vi "ActionVIOnCompile.vi"(8 "error in":errorcluster, 11 "Device Item Ref in":T1 format="%.0x") -> (0 "error out":errorcluster)   [LabVIEW 2024, in "AIM ARINC 429 System Explorer.lvlib"]
uses:
  AIM ARINC 429 System Explorer.lvlib
  <vilib>/NI VeriStand/Custom Device API/Custom Device API.lvlib
  Includes/AIM ARINC 429 Engine.lvlibp/Engine/Custom Device/Inline Execution Unit Compiled Information.ctl
  Includes/AIM ARINC 429 Engine.lvlibp/Engine/Custom Device/Asynchronous Execution Unit Compiled Information.ctl
  Includes/AIM ARINC 429 Engine.lvlibp/Engine/Custom Device/Compiled.Settings.ctl
  Shared/Constants.vi
  Shared/AIM ARINC 429 Shared.lvlib
  Includes/AIM ARINC 429 Engine.lvlibp/Engine/Implementation/Execution Unit Factory/Execution Unit Factory.lvclass
  Includes/AIM ARINC 429 Engine.lvlibp/Engine/Implementation/Shared Resources Factory/Shared Resources Factory.lvclass
  Includes/AIM ARINC 429 Engine.lvlibp/Engine/Interfaces/Execution Unit Factory/Execution Unit Factory.lvclass
  Includes/AIM ARINC 429 Engine.lvlibp/Engine/Interfaces/Shared Resources Factory/Shared Resources Factory.lvclass
  Includes/AIM ARINC 429 Engine.lvlibp/1abvi3w/vi.lib/NI VeriStand/Custom Device API/Data Reference.ctl
  Includes/AIM ARINC 429 Engine.lvlibp/1abvi3w/vi.lib/NI VeriStand/Custom Device API/Block Data Reference.ctl
  <vilib>/NI VeriStand/Custom Device API/Set Item Property (Variant).vi
  <vilib>/NI VeriStand/Custom Device API/Custom Device Item Ref.ctl
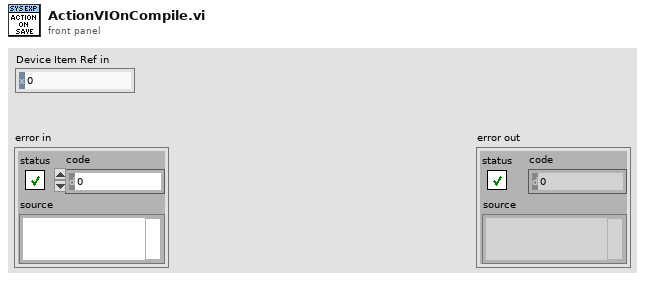
[diagram p1: front panel]
types:
  T1 = typedef "Custom Device API.lvlib/Custom Device Item Ref.ctl" = u64
  T2 = typedef "AIM ARINC 429 System Explorer.lvlibp/Custom Device API.lvlib/Custom Device Item Ref.ctl" = u64
  T3 = typedef "AIM ARINC 429 Engine.lvlibp/Custom Device.lvlib/Compiled.Settings.ctl" = cluster{"Name":string, "Inline Execution Unit Compiled Information":T4[], "Asynchronous Execution Unit Compiled Information":T7[], "Flattened Shared Resources":string}
  T4 = typedef "AIM ARINC 429 Engine.lvlibp/Custom Device.lvlib/Inline Execution Unit Compiled Information.ctl" = cluster{"Flattened Execution Unit":string, "Incoming Buffer":dbl[], "Outgoing Buffer":dbl[], "Incoming Data References":T5[], "Outgoing Data References":T6[]}
  T5 = typedef "AIM ARINC 429 Engine.lvlibp/Custom Device API.lvlib/Data Reference.ctl" = i32
  T6 = typedef "AIM ARINC 429 Engine.lvlibp/Custom Device API.lvlib/Block Data Reference.ctl" = cluster{"Data Reference":T5, "Offset":u64, "Length":u64}
  T7 = typedef "AIM ARINC 429 Engine.lvlibp/Custom Device.lvlib/Asynchronous Execution Unit Compiled Information.ctl" = cluster{"Flattened Execution Unit":string, "Incoming Channel Group Name":string, "Outgoing Channel Group Name":string, "ReadWrite Channel Group Name":string}
  T8 = typedef "Custom Device API.lvlib/Custom Device Item Info.ctl" = cluster{"Name":string, "Is Channel":bool, "GUID":string, "Is Waveform":bool}
  T9 = typedef "AIM ARINC 429 Engine.lvlibp/Interfaces.lvlib/Execution Unit Information.ctl" = cluster{"Execution Unit":refnum<class "Execution Unit.lvclass">, "Incoming Channels":T10[], "Outgoing Channels":T10[], "ReadWrite Channels":T10[]}
  T10 = typedef "AIM ARINC 429 Engine.lvlibp/Custom Device API.lvlib/Custom Device Item Ref.ctl" = u64
  T11 = typedef "AIM ARINC 429 Shared.lvlib/Inline Execution Unit Compiled Information.ctl" = cluster{"Flattened Execution Unit":string, "Incoming Buffer":dbl[], "Outgoing Buffer":dbl[], "Incoming Data References":T12[], "Outgoing Data References":T13[]}
  T12 = typedef "Custom Device API.lvlib/Data Reference.ctl" = i32
  T13 = typedef "Custom Device API.lvlib/Block Data Reference.ctl" = cluster{"Data Reference":T12, "Offset":u64, "Length":u64}
  T14 = typedef "AIM ARINC 429 Shared.lvlib/Asynchronous Execution Unit Compiled Information.ctl" = cluster{"Flattened Execution Unit":string, "Incoming Channel Group Name":string, "Outgoing Channel Group Name":string, "ReadWrite Channel Group Name":string}
  T15 = cluster{"Compiled Grouped Asynchronous Execution Units":T14[]}[]
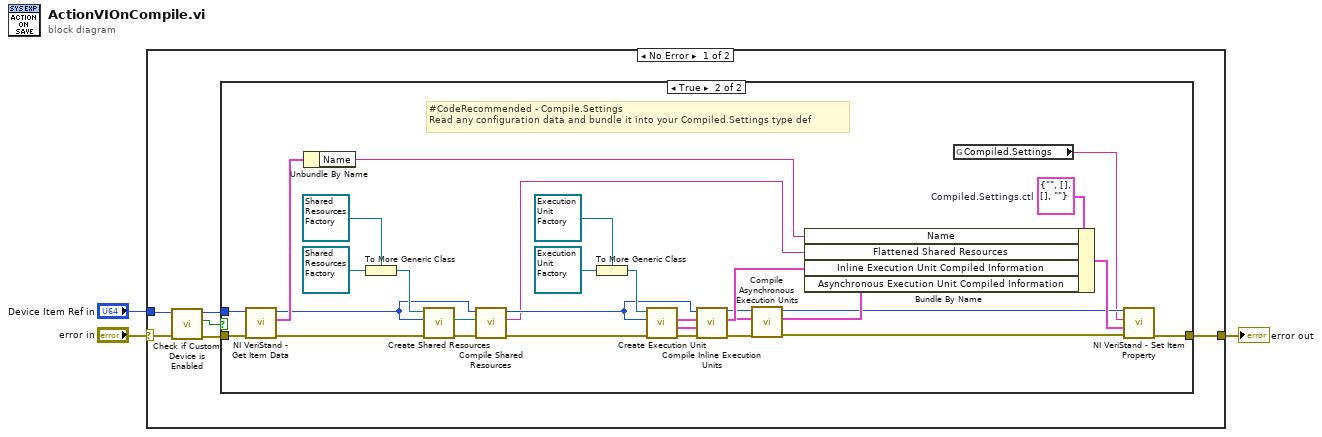
[diagram p0: block diagram]
diagram:
  n1 = case shown="No Error" "error in" {
    selector: "error in" -> [w8 w41]
    tunnel: [w9 w41] -> w2
    tunnel: "Device Item Ref in" -> [w6 _]
    frame No Error {
      n2 = call "Check if Custom Device is Enabled.vi"("error in (no error)"=w8, "AIM ARINC 429 ref"=w6) -> ("error out"=w7:errorcluster, "Custom Device is Enabled"=w4:bool, "AIM ARINC 429 ref"=w5:T2)  [unwired: 7 in]
      n3 = case shown="True" w4 {
        tunnel: [w10 w39] -> w9
        tunnel: w7 -> [w10 w37]
        tunnel: w5 -> [_ w34]
        frame False {
        }
        frame True {
          w12 = T3 {"Name"="", "Inline Execution Unit Compiled Information"=[], "Asynchronous Execution Unit Compiled Information"=[], "Flattened Shared Resources"=""}  # Compiled.Settings.ctl
          # "#CodeRecommended - Compile.Settings\nRead any configuration data and bundle it into your Compiled.Settings type def"
          n4 = call <vilib>:"NI VeriStand - Get Item Data.vi"("error in (no error)"=w37, "Item Ref in"=w34) -> ("error out"=w22:errorcluster, "Item Info"=w38:T8, "Item Ref out"=w18:T1)  [unwired: 6 in, 1 out]
          n5 = Unbundle By Name(w38) -> ("Name"=w35:string)
          n6 = To More Generic Class(target class=refnum<class "Shared Resources Factory.lvclass"> refnum ("Communication Bus Template Interfaces:Interfaces.lvlib:Shared Resources Factory.lvclass"), reference=refnum<class "Shared Resources Factory.lvclass"> refnum ("Shared Resources Factory in")) -> (generic class reference=w19:refnum<class "Shared Resources Factory.lvclass">)
          n7 = call-dynamic "Create Shared Resources.vi"("error in"=w22, "custom device ref"=w18, "shared resources factory in"=w19) -> ("error out"=w17:errorcluster, "shared resources"=w14:refnum<class "Shared Resources.lvclass">)  [unwired: 6 in, 1 out]
          n8 = call "Compile Shared Resources.vi"("error in"=w17, "shared resources"=w14, "device ref in"=w18) -> ("error out"=w16:errorcluster, "flattened shared resources"=w13:string, "device ref out"=w15:T1)  [unwired: 6 in]
          n9 = To More Generic Class(target class=refnum<class "Execution Unit Factory.lvclass"> refnum ("Communication Bus Template Interfaces:Interfaces.lvlib:Execution Unit Factory.lvclass"), reference=refnum<class "Execution Unit Factory.lvclass"> refnum ("Communication Bus Template Interfaces:Implementation.lvlib:Execution Unit Factory.lvclass")) -> (generic class reference=w33:refnum<class "Execution Unit Factory.lvclass">)
          n10 = call-dynamic "Create Execution Unit.vi"("error in"=w16, "Item Ref"=w15, "Execution Unit Factory in"=w33) -> ("error out"=w36:errorcluster, "Asynchronous Execution Units"=w25:T9[], "Inline Execution Units"=w31:T9[])  [unwired: 5 in, 1 out]
          n11 = call "Compile Inline Execution Units.vi"("error in"=w36, "Inline Execution Units"=w31, "Device Ref in"=w15) -> ("error out"=w30:errorcluster, "Compiled Inline Execution Units"=w32:T11[], "Device Ref out"=w29:T1)  [unwired: 6 in]
          n12 = call "Compile Asynchronous Execution Units.vi"("Device Ref in"=w29, "Asynchronous Execution Units"=w25, "error in"=w30) -> ("Device Ref out"=w26:T1, "Compiled Asynchronous Execution Units"=w28:T15, "error out"=w27:errorcluster)  [unwired: 5 in]
          n13 = Bundle By Name(cluster=w12, "Name"=w35, "Flattened Shared Resources"=w13, "Inline Execution Unit Compiled Information"=w32, "Asynchronous Execution Unit Compiled Information"=w28) -> (w40:T3)
          n14 = global read "Constants.vi" "Compiled.Settings"() -> (w11:string)
          n15 = call-poly <vilib>:"NI VeriStand - Set Item Property.vi"("error in (no error)"=w27, "Value"=w40, "Property Name"=w11, "Item Ref in"=w26) -> ("error out"=w39:errorcluster)  [unwired: 5 in, 2 out]
        }
      }
    }
    frame Error {
    }
  }
  "error out" <- w2
